vi "Create Digital Input.vi"(8 "error in (no error)":errorcluster, 10 "Params":variant, 11 "NI Digital Input in":refnum<class "NI Digital Input.lvclass">) -> (0 "error out":errorcluster, 3 "NI Digital Input out":refnum<class "NI Digital Input.lvclass">)   [LabVIEW 2020, in "NI DAQmx.lvlib" / "NI Digital Input.lvclass"]
uses:
  NI Digital Input.lvclass
  D:/WSGitHub/RTFWK/Realization/NI DAQmx Base/NI DAQmx Base.lvclass
  <vilib>/DAQmx/create/channels.llb/DAQmx Create Channel (DI-Digital Input).vi
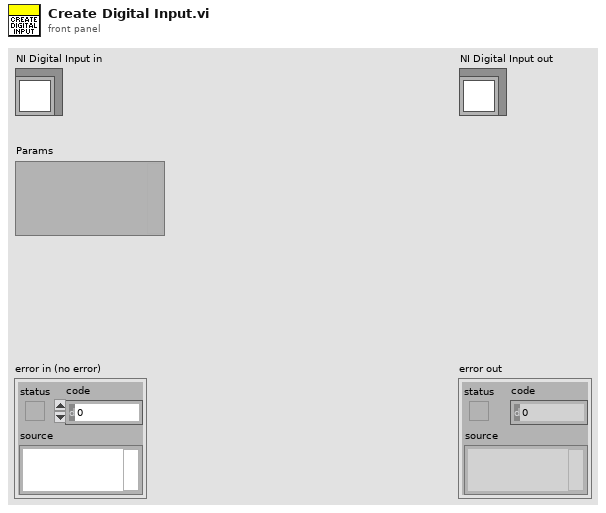
[diagram p1: front panel]
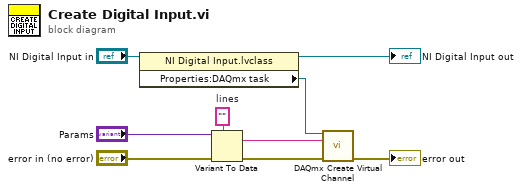
[diagram p0: block diagram]
diagram:
  w6 = ""  # lines
  n1 = property class="NI Digital Input.lvclass"(reference="NI Digital Input in") -> (reference out=→"NI Digital Input out":refnum<class "NI Digital Input.lvclass">, "Properties:DAQmx task"=w7:refnum<k21>)  [unwired: 1 in, 1 out]
  n2 = Variant To Data(error in="error in (no error)", type=w6, Variant="Params") -> (data=w2:string, error out=w3:errorcluster)
  n3 = call-poly <vilib>:"DAQmx Create Virtual Channel.vi"("task in"=w7, "lines"=w2, "error in"=w3) -> ("error out"=→"error out":errorcluster)  [unwired: 11 in, 1 out]
